vi "Copy .LLB to NI VeriStand dir.vi"(5 "Files Generated by Build":path[](array[path]), 6 "Top Level/Always Included VIs":path[](array[path]), 7 "Destination Path":path, 8 "error in (no error)":errorcluster, 9 "Target Name":string, 10 "Build Specification Name":string, 11 "Project Path":path) -> (0 "error out":errorcluster)   [LabVIEW 2024]
doc: "This VI is called after each run of a build specification. The VI will copy the generated LLB (Engine or System Explorer) into the VeriStand Custom Device folder (...\\Documents\\National Instruments\\NI VeriStand 2013...)."
uses:
  NationalInstruments.VeriStand
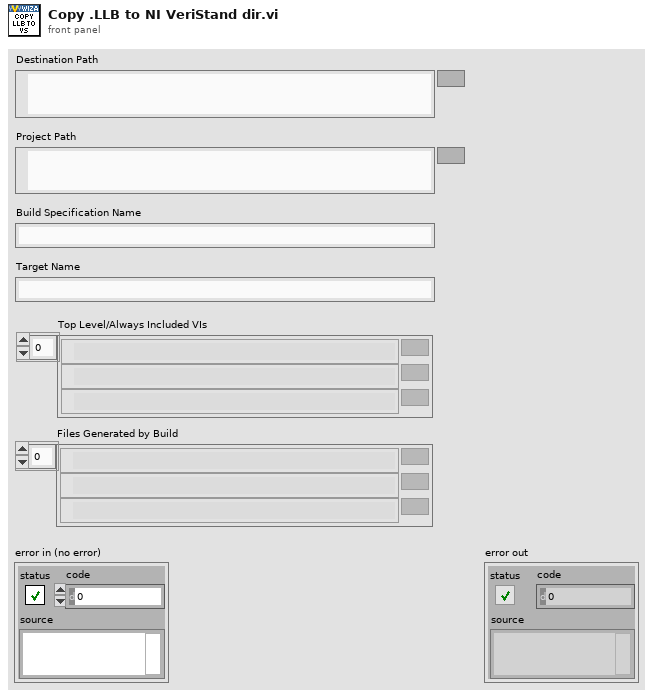
[diagram p1: front panel]
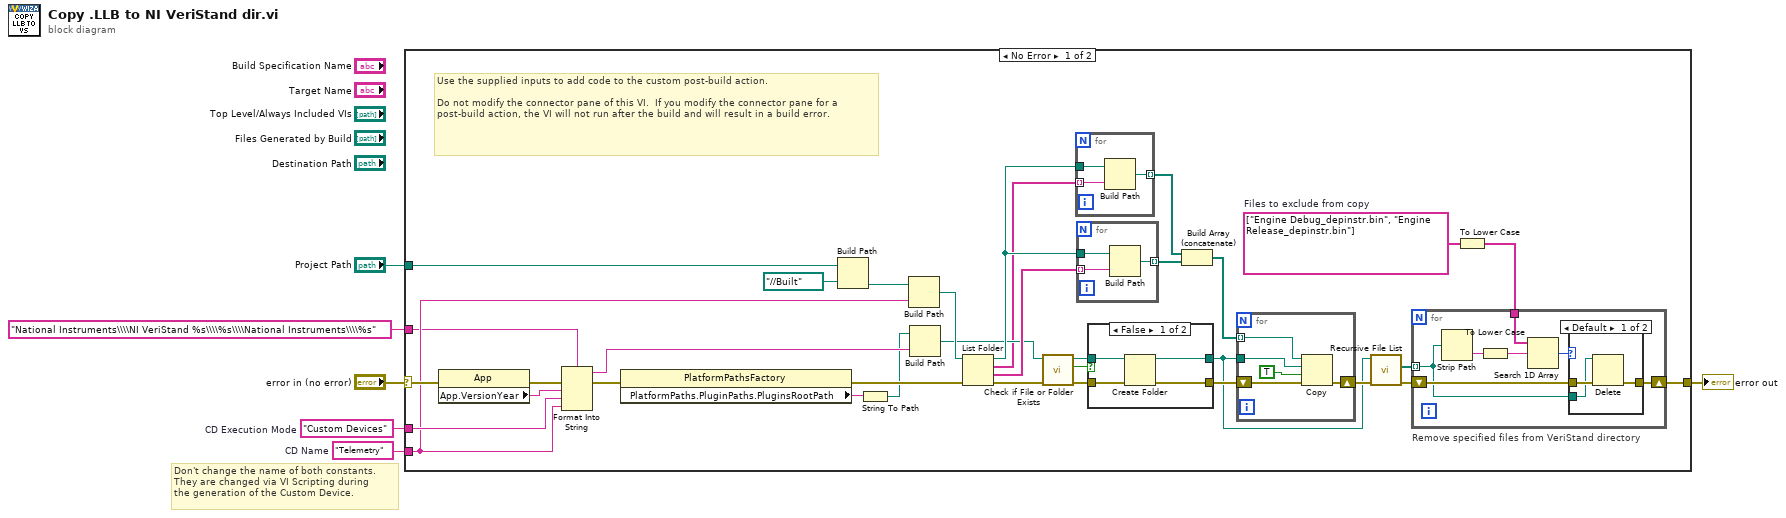
[diagram p0: block diagram]
diagram:
  w3 = "Telemetry"  # CD Name
  w4 = "Custom Devices"  # CD Execution Mode
  # "Don't change the name of both constants.\nThey are changed via VI Scripting during\nthe generation of the Custom Device."
  n1 = case shown="No Error" "error in (no error)" {
    selector: "error in (no error)" -> [w24 w69]
    tunnel: [w12 w69] -> w2
    tunnel: "Project Path" -> [w21 _]
    tunnel: w4 -> [w25 _]
    tunnel: w3 -> [w23 _]
    tunnel: "National Instruments\\\\NI VeriStand %s\\\\%s\\\\National Instruments\\\\%s" ("name or relative path") -> [w11 _]
    frame No Error {
      w18 = string[] ["Engine Debug_depinstr.bin", "Engine Release_depinstr.bin"]  # Files to exclude from copy
      # "Use the supplied inputs to add code to the custom post-build action.\n\nDo not modify the connector pane of this VI.  If you modify the connector pane for a post-build action, the VI will not run after the build and will result in a build error."
      n2 = property class="App"(error in=w24) -> (error out=w28:errorcluster, "App.VersionYear"=w27:string)  [unwired: 1 in, 1 out]
      n3 = Format Into String(format string=w11, error in=w28, w27, w25, w23) -> (resulting string=w29:string, error out=w9:errorcluster)  [unwired: 1 in]
      n4 = property class="PlatformPathsFactory"(error in=w9) -> (error out=w10:errorcluster, "PlatformPaths.PluginPaths.PluginsRootPath"=w8:string)  [unwired: 1 in, 1 out]
      n5 = Build Path(base path=w21, name or relative path=path "../../Built") -> (appended path=w30:path)
      n6 = String To Path(string=w8) -> (path=w7:path)
      n7 = Build Path(base path=w30, name or relative path=w23) -> (appended path=w32:path)
      n8 = Build Path(base path=w7, name or relative path=w29) -> (appended path=w26:path)
      n9 = List Folder(path=w32, error in=w10) -> (path out=w34:path, filenames=w19:string[], folder names=w35:string[], error out=w31:errorcluster)  [unwired: 2 in]
      n10 = call <vilib>:"Check if File or Folder Exists.vi"("error in (no error)"=w31, "path"=w26) -> ("error out"=w36:errorcluster, "file or folder exists?"=w38:bool, "dup path"=w37:path)  [unwired: 7 in]
      n11 = for {
        tunnel: w19 -> [w67] mode=indexing
        tunnel: w34 -> [w68]
        tunnel: [w66] -> w40 mode=indexing
        n12 = Build Path(base path=w68, name or relative path=w67) -> (appended path=w66:path)
      }
      n13 = for {
        tunnel: w35 -> [w64] mode=indexing
        tunnel: w34 -> [w65]
        tunnel: [w63] -> w33 mode=indexing
        n14 = Build Path(base path=w65, name or relative path=w64) -> (appended path=w63:path)
      }
      n15 = case shown="False" w38 {
        tunnel: w37 -> [w55 w57]
        tunnel: w36 -> [w54 w56]
        tunnel: [w53 w57] -> w13
        tunnel: [w52 w56] -> w20
        frame False {
          n16 = Create Folder(path (use dialog)=w55, error in=w54) -> (created path=w53:path, error out=w52:errorcluster)  [unwired: 1 in, 1 out]
        }
        frame True {
        }
      }
      n17 = Build Array (concatenate)(w40, w33) -> (w39:path[])
      n18 = for {
        tunnel: w39 -> [w59] mode=indexing
        shift-right: [w60] -> w14
        shift-left: w20 -> [w61]
        tunnel: w13 -> [w58]
        n19 = Copy(8:w61, 9:TRUE ("overwrite (F)"), 10:w58, 11:w59) -> (0:w60:errorcluster)  [unwired: 1 in, 2 out]
      }
      n20 = call <vilib>:"Recursive File List.vi"("error in (no error)"=w14, "Folder Path"=w13) -> ("error out"=w17:errorcluster, "All Files in Dir"=w16:path[])  [unwired: 5 in, 3 out]
      n21 = To Lower Case(string=w18) -> (all lower case string=w15:string[])
      n22 = for "Remove specified files from VeriStand directory" {
        shift-right: [w42] -> w12
        shift-left: w17 -> [w44]
        tunnel: w16 -> [w41] mode=indexing
        tunnel: w15 -> [w45]
        n23 = Strip Path(path=w41) -> (name=w47:string)  [unwired: 1 out]
        n24 = To Lower Case(string=w47) -> (all lower case string=w46:string)
        n25 = Search 1D Array(1D array=w45, element=w46) -> (index of element=w43:i32)  [unwired: 1 in]
        n26 = case shown="Default" w43 {
          tunnel: w44 -> [w50 w51]
          tunnel: [w49 w51] -> w42
          tunnel: w41 -> [w48 _]
          frame Default {
            n27 = Delete(path (use dialog)=w48, error in=w50) -> (error out=w49:errorcluster)  [unwired: 3 in, 2 out]
          }
          frame -1 {
          }
        }
      }
    }
    frame Error {
    }
  }
  "error out" <- w2
